vi "USRP Signal Generator.vi"() -> ()   [LabVIEW 2021]
uses:
  <vilib>/addons/Modulation/Analog/controls/Complex Data Waveform.ctl
  <vilib>/measure/maspectr.llb/Power Spectrum and PSD Export Mode.ctl
  <vilib>/Analysis/1siggen.llb/Ramp Pattern by Samples.vi
  system stop.vi
  <vilib>/measure/matone.llb/Extract Single Tone Information 1 Chan (CDB).vi
  <vilib>/measure/maspectr.llb/FFT Power Spectrum and PSD for 1 Chan (CDB).vi
  <instrlib>/niUSRP/niUSRP Write Tx Data (CDB Cluster).vi
  <instrlib>/niUSRP/niUSRP Fetch Rx Data (CDB Cluster).vi
  <vilib>/addons/Modulation/niAMT.lvlib
  <vilib>/measure/NI_MAPro.lvlib
  <vilib>/Analysis/NI_AALBase.lvlib
  <vilib>/Analysis/NI_AALPro.lvlib
panel:
  out "Threshold count":i32
  out "Threshold indices":i32[](array[numeric])
  out "detected Amplitude":dbl format="%.2p"
  out "detected frequency":dbl format="%.2p"
  out "Tx Waveform Graph":dbl[](graph)
  in  "Frequency":dbl format="%#_13g"
  in  "Duration":dbl format="%#_13g"
  in  "number of samples Rx on USRP":i64=100000
  in  "stop":bool
  out "Received Waveform Graph":cluster{"f0":dbl, "df":dbl, "magnitude":dbl[]}(graph)
  out "coerced IQ rate":dbl=100000.0 format="%#_6p"
  out "coerced carrier frequency":dbl=100000.0 format="%#_6p"
  in  "gain Rx":dbl format="%#_6f"
  in  "device names Rx":refnum<k15>
  in  "gain Tx":dbl format="%#_6f"
  in  "carrier frequency":dbl=100000.0 format="%#_6p"
  in  "IQ rate":dbl=100000.0 format="%#_6p"
  in  "device names Tx":refnum<k15>
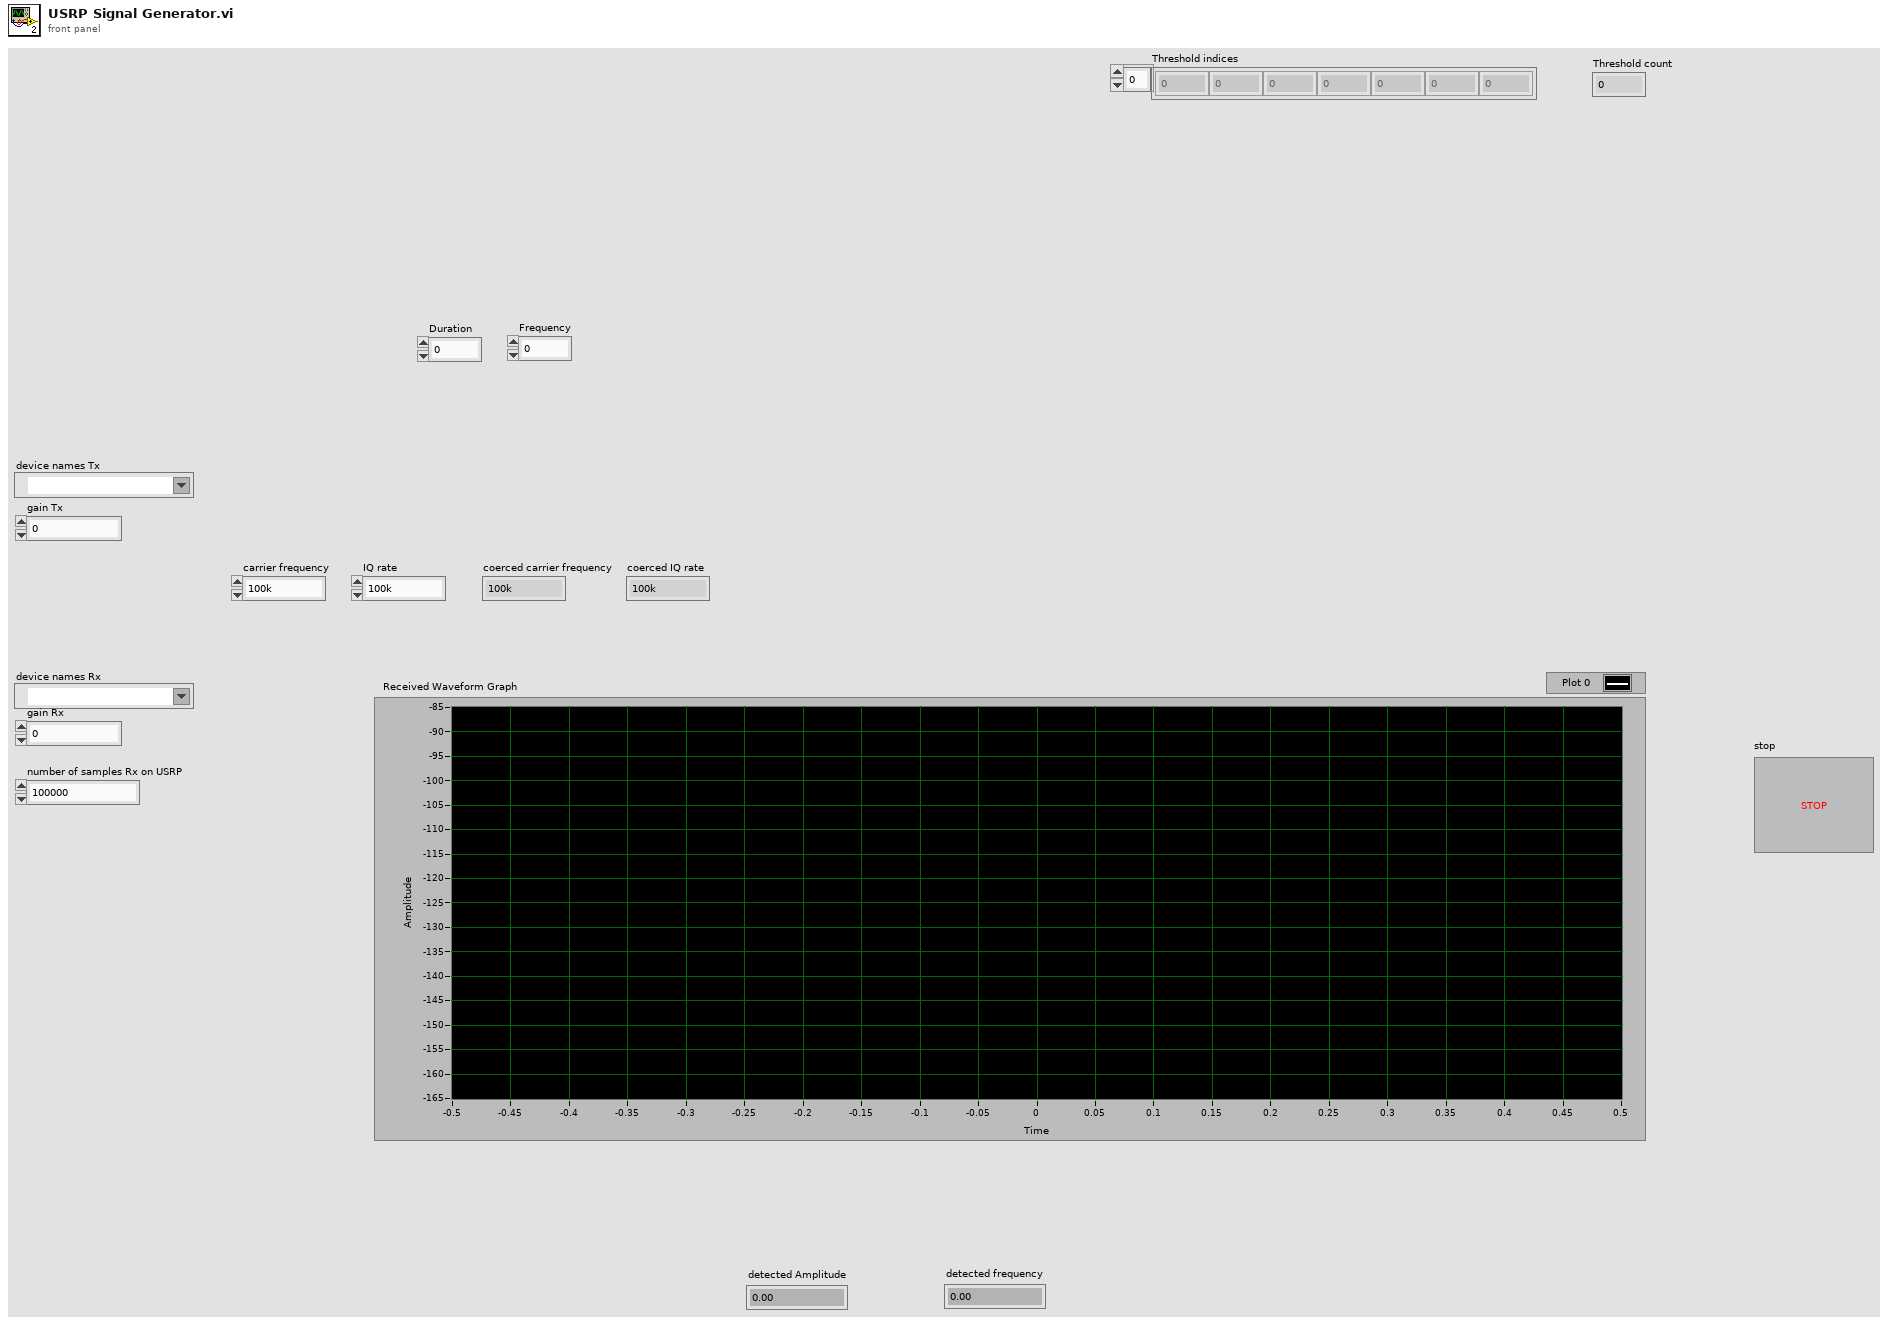
[diagram p1: front panel]
types:
  T1 = typedef "niAMT.lvlib/Complex Data Waveform.ctl" = cluster{"t0":dbl, "dt":dbl, "Y":cdb[]}
  T2 = typedef "NI_MAPro.lvlib/Power Spectrum and PSD Export Mode.ctl" = u16
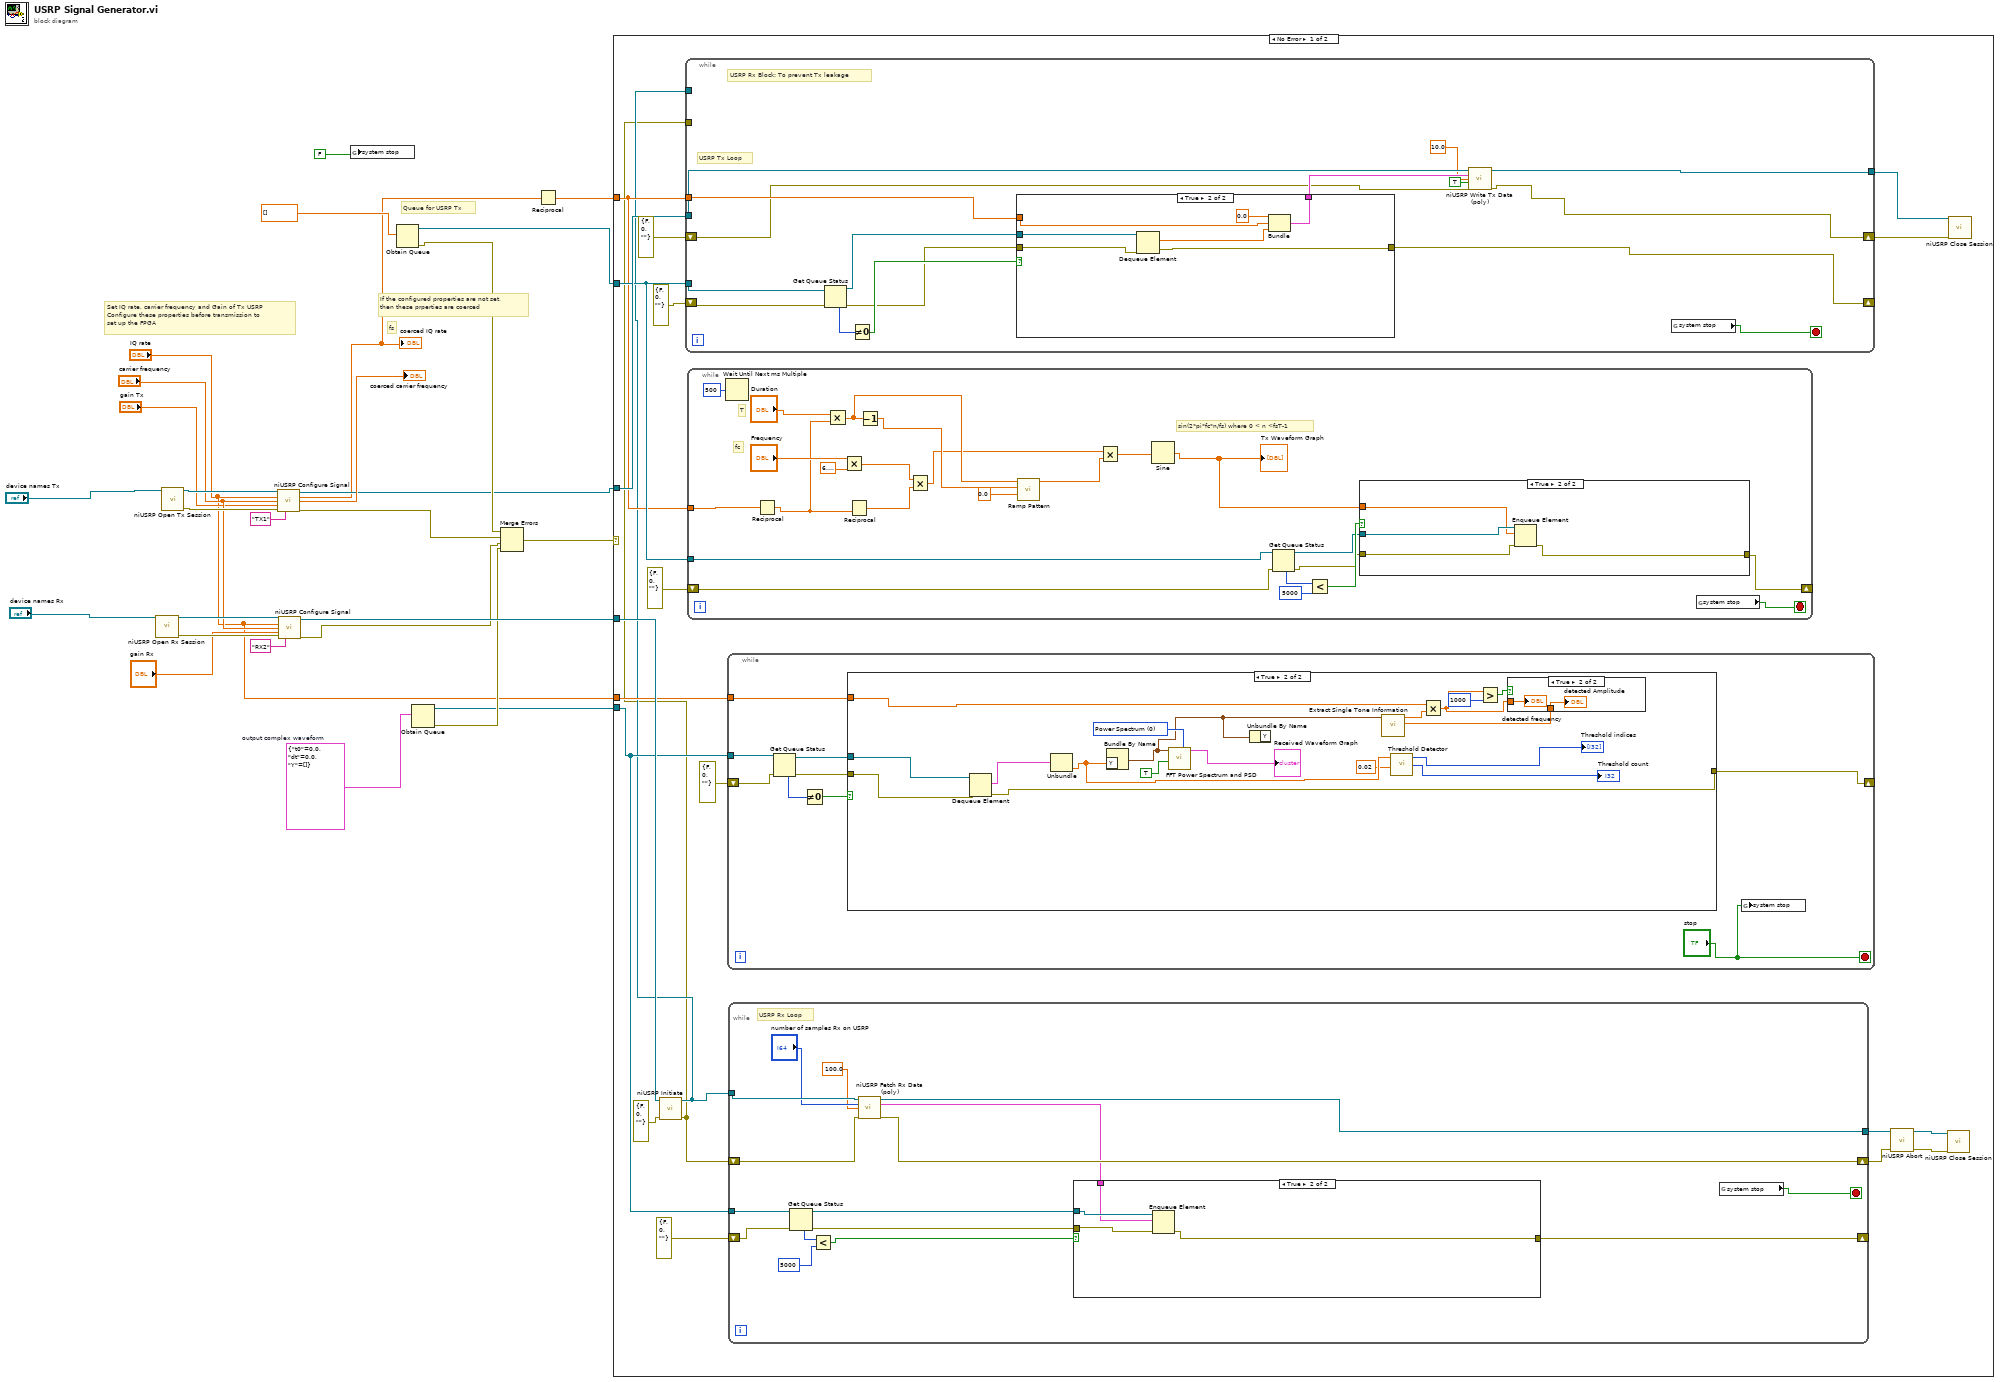
[diagram p0: block diagram]
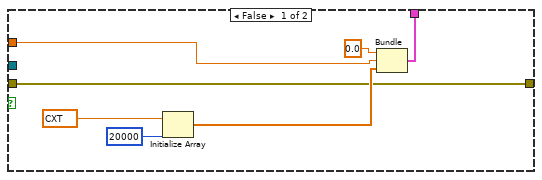
[diagram p6: hidden frame]
diagram:
  w10 = T1 {"t0"=0.0, "dt"=0.0, "Y"=[]}  # output complex waveform
  # "fs"
  # "If the configured properties are not set,\nthen these prperties are coerced"
  # "Set IQ rate, carrier frequency and Gain of Tx USRP\nConfigure these properties before transmission to\nset up the FPGA"
  # "Queue for USRP Tx"
  n1 = call <instrlib>:"niUSRP Open Rx Session.vi"("device names"="device names Rx") -> ("session handle out"=w23:refnum<k15>, "error out"=w22:errorcluster)  [unwired: 13 in]
  n2 = call <instrlib>:"niUSRP Open Tx Session.vi"("device names"="device names Tx") -> ("session handle out"=w26:refnum<k15>, "error out"=w25:errorcluster)  [unwired: 13 in]
  n3 = call <instrlib>:"niUSRP Configure Signal.vi"("session handle"=w26, "IQ rate"="IQ rate", "carrier frequency"="carrier frequency", "gain"="gain Tx", "error in (no error)"=w25, "active antenna"="TX1") -> ("session handle out"=w11:refnum<k15>, "coerced IQ rate"=w5:dbl, "coerced carrier frequency"=→"coerced carrier frequency":dbl, "error out"=w17:errorcluster)  [unwired: 5 in, 1 out]
  "coerced IQ rate" <- w5
  n4 = call <instrlib>:"niUSRP Configure Signal.vi"("session handle"=w23, "IQ rate"="IQ rate", "carrier frequency"="carrier frequency", "gain"="gain Rx", "error in (no error)"=w22, "active antenna"="RX2") -> ("session handle out"=w12:refnum<k15>, "error out"=w9:errorcluster)  [unwired: 5 in, 3 out]
  n5 = global write "system stop.vi" "system stop"(FALSE) -> ()
  n6 = Obtain Queue(element data type=dbl[] []) -> (queue out=w6:refnum<queue>, error out=w15:errorcluster)  [unwired: 4 in, 1 out]
  n7 = Obtain Queue(element data type=w10) -> (queue out=w7:refnum<queue>, error out=w8:errorcluster)  [unwired: 4 in, 1 out]
  n8 = Merge Errors(w15, w17, w9, w8) -> (w14:errorcluster)
  n9 = Reciprocal(x=w5) -> (1/x=w4:dbl)
  n10 = case shown="No Error" w14 {
    tunnel: w12 -> [w39 _]
    tunnel: w11 -> [w38 _]
    tunnel: w7 -> [w36 _]
    tunnel: w6 -> [w33 _]
    tunnel: w4 -> [w31 _]
    tunnel: "IQ rate" -> [w30 _]
    frame No Error {
      n11 = call <instrlib>:"niUSRP Initiate.vi"("session handle"=w39, "error in (no error)"=errorcluster {"status"=FALSE, "code"=0, "source"=""}) -> ("session handle out"=w29:refnum<k15>, "error out"=w28:errorcluster)  [unwired: 12 in]
      n12 = while {
        shift-right: [w130] -> w46
        shift-left: errorcluster {"status"=FALSE, "code"=0, "source"=""} ("error in (no error)") -> [w131]
        tunnel: [w143] -> w45
        tunnel: w38 -> [w141]
        tunnel: w33 -> [w140]
        shift-right: [w134] -> _
        shift-left: errorcluster {"status"=FALSE, "code"=0, "source"=""} ("error in (no error)") -> [w139]
        tunnel: w31 -> [w133]
        tunnel: w29 -> [_]
        tunnel: w28 -> [_]
        stop <- w142 stop-if-true
        # "USRP Rx Block: To prevent Tx leakage"
        # "USRP Tx Loop"
        n13 = Get Queue Status(queue=w140, error in (no error)=w139) -> (queue out=w136:refnum<queue>, error out=w135:errorcluster, # elements in queue=w138:i32)  [unwired: 1 in, 5 out]
        n14 = Not Equal To 0?(x=w138) -> (x != 0?=w137:bool)
        n15 = case shown="True" w137 {
          tunnel: w136 -> [_ w157]
          tunnel: w135 -> [w144 w156]
          tunnel: [w144 w155] -> w134
          tunnel: w133 -> [w146 w153]
          tunnel: [w145 w151] -> w132
          frame False {
            n16 = Initialize Array(cxt 0.0+0.0i, 20000) -> (w148:cxt[])
            n17 = Bundle(0.0, w146, w148) -> (w145:cluster{dbl, dbl, cxt[]})  [unwired: 1 in]
          }
          frame True {
            n18 = Dequeue Element(queue=w157, error in (no error)=w156) -> (element=w154:dbl[], error out=w155:errorcluster)  [unwired: 1 in, 2 out]
            n19 = Bundle(0.0, w153, w154) -> (w151:cluster{dbl, dbl, dbl[]})  [unwired: 1 in]
          }
        }
        n20 = call-poly <instrlib>:"niUSRP Write Tx Data (poly).vi"("session handle"=w141, "data"=w132, "timeout"=10.0, "end of data?"=TRUE, "error in (no error)"=w131) -> ("session handle out"=w143:refnum<k15>, "error out"=w130:errorcluster)  [unwired: 9 in]
        n21 = global read "system stop.vi" "system stop"() -> (w142:bool)
      }
      n22 = while {
        tunnel: w33 -> [w60]
        shift-right: [w54] -> _
        shift-left: errorcluster {"status"=FALSE, "code"=0, "source"=""} ("error in (no error)") -> [w61]
        tunnel: w31 -> [w50]
        stop <- w52 stop-if-true
        # "T"
        # "fc"
        # "sin(2*pi*fc*n/fs) where 0 < n <fsT-1"
        n23 = Wait Until Next ms Multiple(millisecond multiple=500) -> ()  [unwired: 1 out]
        n24 = Reciprocal(x=w50) -> (1/x=w49:dbl)
        n25 = Multiply(x="Duration", y=w49) -> (x*y=w66:dbl)
        n26 = Multiply(x="Frequency", y=6.283185307179586) -> (x*y=w68:dbl)
        n27 = Reciprocal(x=w49) -> (1/x=w51:dbl)
        n28 = Decrement(x=w66) -> (x-1=w67:dbl)
        n29 = Multiply(x=w68, y=w51) -> (x*y=w63:dbl)
        n30 = call-poly <vilib>:"Ramp Pattern.vi"("start"=0.0, "end"=w67, "samples"=w66) -> ("Ramp Pattern"=w64:dbl[])  [unwired: 7 in, 1 out]
        n31 = Multiply(x=w63, y=w64) -> (x*y=w62:dbl[])
        n32 = Sine(x=w62) -> (sin(x)=w53:dbl[])
        "Tx Waveform Graph" <- w53
        n33 = Get Queue Status(queue=w60, error in (no error)=w61) -> (queue out=w56:refnum<queue>, error out=w55:errorcluster, # elements in queue=w59:i32)  [unwired: 1 in, 5 out]
        n34 = Less?(x=w59, y=5000) -> (x < y?=w57:bool)
        n35 = case shown="True" w57 {
          tunnel: w56 -> [_ w76]
          tunnel: w55 -> [w72 w75]
          tunnel: [w72 w74] -> w54
          tunnel: w53 -> [_ w73]
          frame False {
          }
          frame True {
            n36 = Enqueue Element(queue=w76, element=w73, error in (no error)=w75) -> (error out=w74:errorcluster)  [unwired: 1 in, 2 out]
          }
        }
        n37 = global read "system stop.vi" "system stop"() -> (w52:bool)
      }
      n38 = while {
        tunnel: w36 -> [w85]
        shift-right: [w79] -> _
        shift-left: errorcluster {"status"=FALSE, "code"=0, "source"=""} ("error in (no error)") -> [w84]
        tunnel: w30 -> [w77]
        stop <- "stop" stop-if-true
        n39 = Get Queue Status(queue=w85, error in (no error)=w84) -> (queue out=w83:refnum<queue>, error out=w82:errorcluster, # elements in queue=w80:i32)  [unwired: 1 in, 5 out]
        n40 = Not Equal To 0?(x=w80) -> (x != 0?=w81:bool)
        n41 = case shown="True" w81 {
          tunnel: w83 -> [_ w102]
          tunnel: w82 -> [w86 w101]
          tunnel: [w86 w104] -> w79
          tunnel: w77 -> [_ w103]
          frame False {
          }
          frame True {
            w97 = T2 0 items=["Power Spectrum", "Power Spectral Density"] ("export mode")
            n42 = Dequeue Element(queue=w102, error in (no error)=w101) -> (element=w100:T1, error out=w104:errorcluster)  [unwired: 1 in, 2 out]
            n43 = Unbundle(w100) -> ("Y"=w94:cdb[])  [unwired: 2 out]
            n44 = Bundle By Name("Y"=w94) -> (w95:waveform(cdb))  [unwired: 1 in]
            n45 = call-poly <vilib>:"FFT Power Spectrum and PSD.vi"("export mode"=w97, "dB On (F)"=TRUE, "time signal"=w95) -> ("Power Spectrum / PSD"=→"Received Waveform Graph":cluster{"f0":dbl, "df":dbl, "magnitude":dbl[]})  [unwired: 5 in, 3 out]
            n46 = Unbundle By Name(w95) -> ()  [unwired: 1 out]
            n47 = call-poly <vilib>:"Extract Single Tone Information.vi"("time signal in"=w95) -> ("detected amplitude"=w87:dbl, "detected frequency"=w96:dbl)  [unwired: 5 in, 4 out]
            n48 = call <vilib>:"Threshold Detector.vi"("threshold"=0.02, "X"=w94) -> ("count"=→"Threshold count":i32, "Indices"=→"Threshold indices":i32[])  [unwired: 1 in, 1 out]
            n49 = Multiply(x=w103, y=w96) -> (x*y=w88:dbl)
            n50 = Greater?(x=w88, y=1000) -> (0:w89:bool)
            n51 = case shown="True" w89 {
              tunnel: w88 -> [_ w106]
              tunnel: w87 -> [_ w105]
              frame False {
              }
              frame True {
                "detected frequency" <- w106
                "detected Amplitude" <- w105
              }
            }
          }
        }
        n52 = global write "system stop.vi" "system stop"("stop") -> ()
      }
      n53 = while {
        tunnel: w29 -> [w122]
        tunnel: [w120] -> w41
        shift-right: [w119] -> w40
        shift-left: w28 -> [w121]
        tunnel: w36 -> [w116]
        shift-right: [w108] -> _
        shift-left: errorcluster {"status"=FALSE, "code"=0, "source"=""} ("error in (no error)") -> [w115]
        stop <- w118 stop-if-true
        # "USRP Rx Loop"
        n54 = Get Queue Status(queue=w116, error in (no error)=w115) -> (queue out=w114:refnum<queue>, error out=w110:errorcluster, # elements in queue=w113:i32)  [unwired: 1 in, 5 out]
        n55 = Less?(x=w113, y=5000) -> (x < y?=w111:bool)
        n56 = call-poly <instrlib>:"niUSRP Fetch Rx Data (poly).vi"("session handle"=w122, "number of samples"="number of samples Rx on USRP", "timeout"=100.0, "error in (no error)"=w121) -> ("session handle out"=w120:refnum<k15>, "data"=w109:cluster{"t0":dbl, "dt":dbl, "Y":cdb[]}, "error out"=w119:errorcluster)  [unwired: 8 in, 1 out]
        n57 = case shown="True" w111 {
          tunnel: w114 -> [_ w127]
          tunnel: w110 -> [w123 w126]
          tunnel: w109 -> [_ w125]
          tunnel: [w123 w124] -> w108
          frame False {
          }
          frame True {
            n58 = Enqueue Element(queue=w127, element=w125, error in (no error)=w126) -> (error out=w124:errorcluster)  [unwired: 1 in, 2 out]
          }
        }
        n59 = global read "system stop.vi" "system stop"() -> (w118:bool)
      }
      n60 = call <instrlib>:"niUSRP Abort.vi"("session handle"=w41, "error in (no error)"=w40) -> ("session handle out"=w44:refnum<k15>, "error out"=w43:errorcluster)  [unwired: 12 in]
      n61 = call <instrlib>:"niUSRP Close Session.vi"("session handle"=w44, "error in (no error)"=w43) -> ()  [unwired: 13 in, 1 out]
      n62 = call <instrlib>:"niUSRP Close Session.vi"("session handle"=w45, "error in (no error)"=w46) -> ()  [unwired: 13 in, 1 out]
    }
    frame Error {
    }
  }
